vi "ROSSubscriber.vi"(2 "Response":T2, 3 "ROS":T3={"topic port"=1236, "Node"="/labview", "topic"="/robot/head/command_head_nod", "type"="std_msgs/Bool", "node port"=7000, "error "={"status"=FALSE, "code"=0, "source"=""}, "Direction"=enum."Publisher", "Update (ms)"=1, "FIFO size"=1}) -> ()   [LabVIEW 2015]
uses:
  SubVIs/_ROSControl.ctl
  SubVIs/_ROSDirection.ctl
  Console/Servers/ServerSubs/ROSLog.ctl
  _ROSDefinition.vi
panel:
  out "publishers":T1(array[cluster])
  out "Queue log":string
  out "read":string
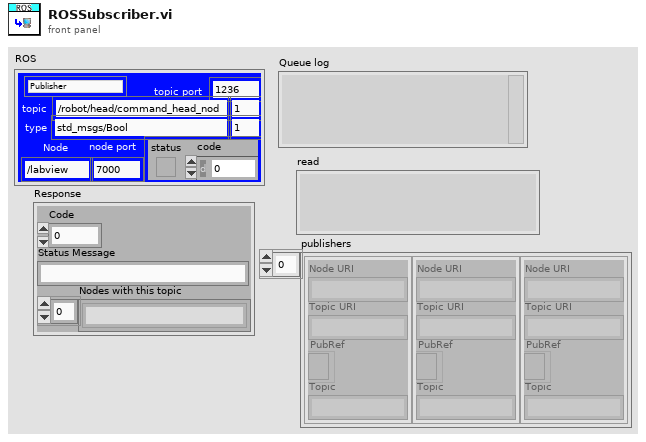
[diagram p1: front panel]
types:
  T1 = cluster{"Node URI":string, "Topic URI":string, "PubRef":refnum<k5>, "Topic":string}[]
  T2 = cluster{"Code":i32, "Status Message":string, "Nodes with this topic":string[]}
  T3 = typedef "_ROSControl.ctl" = cluster{"topic port":u16, "Node":string, "topic":string, "type":string, "node port":u16, "error ":errorcluster, "Direction":T4, "Update (ms)":u16, "FIFO size":u16}
  T4 = typedef "_ROSDirection.ctl" = enum16{"Node", "Publisher", "Subscriber", "ServiceClient", "ServiceProvider"}
  T5 = enum16{"Reset Log", "Add Client", "Remove Client", "Add Task"}
  T6 = cluster{"Node URI":string, "Topic URI":string, "PubRef":refnum<k5>, "Topic":string}
  T7 = typedef "ROSLog.ctl" = cluster{"Sent":string, "Reply":string, "MethodName":string, "success":bool, "Dir1":string, "Dir2":string, "Time Stamp":string, "error":errorcluster, "Preamble":string, "Midamble":string, "Postamble":string}
  T8 = cluster{"Caller ID":string, "Topic Name":string, "Node URIs":string[]}
  T9 = cluster{"Protocol":string, "Code":i32, "IP":string, "Port":i32}
  T10 = cluster{"Protocol":string, "Topic URI":string, "PubRef":refnum<k5>, "topic":string}
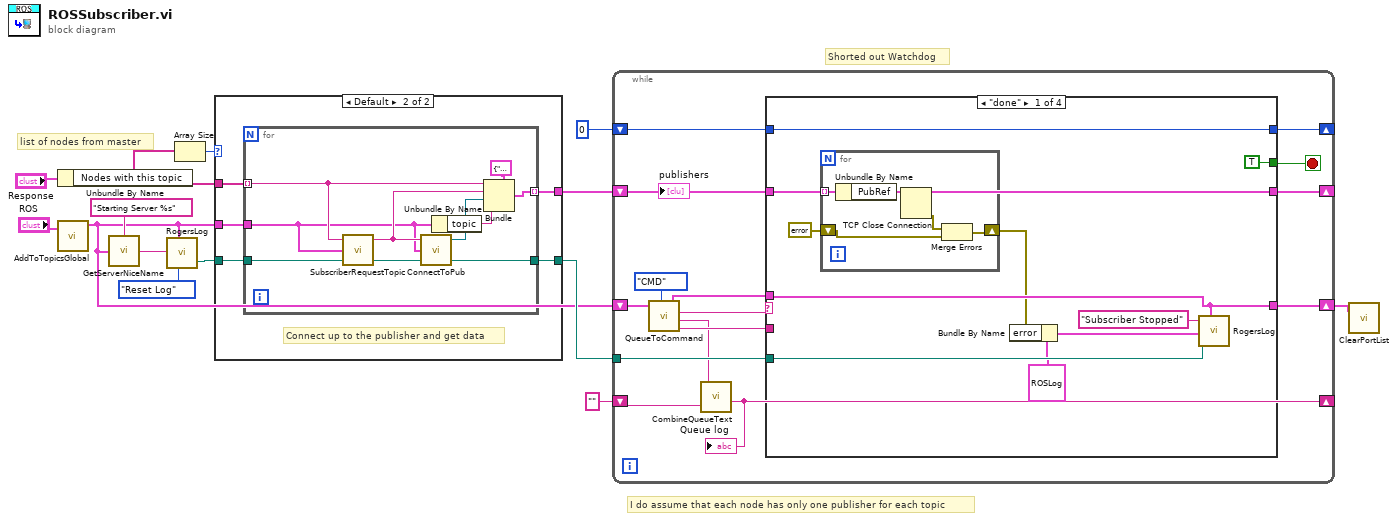
[diagram p0: block diagram]
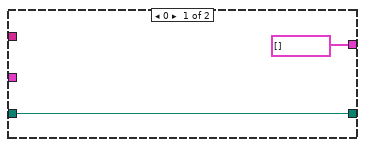
[diagram p2: hidden frame]
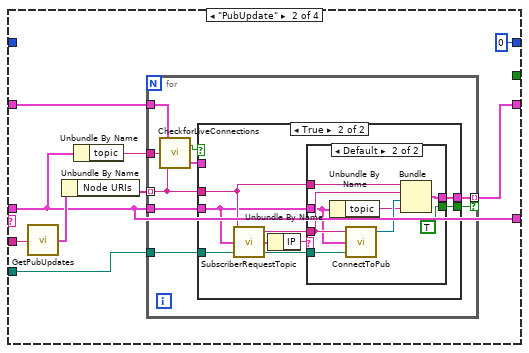
[diagram p3: hidden frame]
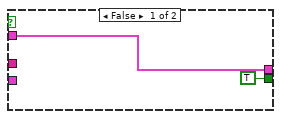
[diagram p4: hidden frame]
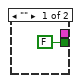
[diagram p5: hidden frame]
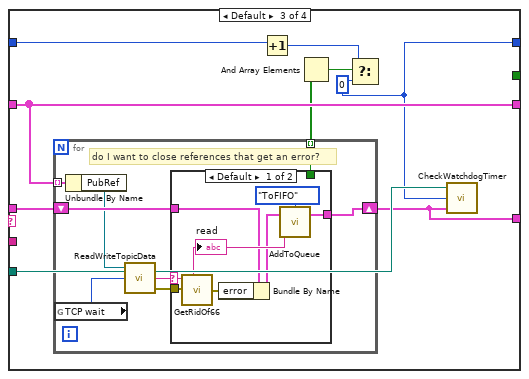
[diagram p6: hidden frame]
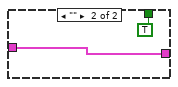
[diagram p7: hidden frame]
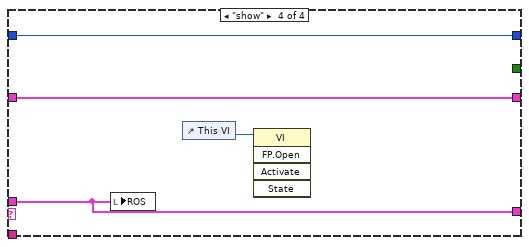
[diagram p8: hidden frame]
diagram:
  # "Shorted out Watchdog"
  # "I do assume that each node has only one publisher for each topic"
  # "list of nodes from master"
  n1 = Unbundle By Name("Response") -> ("Nodes with this topic"=w6:string[])
  n2 = call "AddToTopicsGlobal.vi"("ROS in"="ROS") -> ("ROS out"=w1:T3)  [unwired: 2 in]
  n3 = call "GetServerNiceName.vi"("ROS"=w1, "Text to add"="Starting Server %s") -> ("String"=w11:string)
  n4 = call "RogersLog.vi"("Text to add"=w11, "ROS"=w1, "Task"=T5."Reset Log") -> ("LogPath out"=w9:path)  [unwired: 2 in, 1 out]
  n5 = Array Size(array=w6) -> (size(s)=w5:i32)
  n6 = case shown="Default" w5 {
    tunnel: w6 -> [_ w21]
    tunnel: [T1 [] w20] -> w13
    tunnel: w9 -> [w15 w19]
    tunnel: w1 -> [_ w18]
    tunnel: [w15 w17] -> w8
    frame 0 {
    }
    frame Default {
      # "Connect up to the publisher and get data"
      n7 = for {
        tunnel: w21 -> [w28] mode=indexing
        tunnel: [w25] -> w20 mode=indexing
        tunnel: w19 -> [w31]
        tunnel: w18 -> [w23]
        tunnel: [w29] -> w17
        n8 = call "SubscriberRequestTopic.vi"("LogPath in"=w31, "ROS"=w23, "Node URI"=w28) -> ("LogPath out"=w30:path, "Topic URI"=w27:string)  [unwired: 1 out]
        n9 = call "ConnectToPub.vi"("LogPath in"=w30, "ROS"=w23, "IP"=w27) -> ("LogPath out"=w29:path, "PubRef"=w26:refnum<k5>)  [unwired: 1 out]
        n10 = Unbundle By Name(w23) -> ("topic"=w22:string)
        n11 = Bundle(cluster=T6 {"Node URI"="", "Topic URI"="", "PubRef"=refnum, "Topic"=""} ("output cluster"), "Node URI"=w28, "Topic URI"=w27, "PubRef"=w26, "Topic"=w22) -> (w25:T6)
      }
    }
  }
  n12 = while {
    shift-right: [w42] -> _
    shift-left: w13 -> [w46]
    tunnel: w8 -> [w41]
    shift-right: [w39] -> _
    shift-left: 0 -> [w40]
    shift-right: [w36] -> _
    shift-left: "" ("New List") -> [w38]
    shift-right: [w33] -> w3
    shift-left: w1 -> [w35]
    stop <- w44 stop-if-true
    n13 = call "QueueToCommand.vi"("ROS"=w35, "Check"=enum16{"Cmd+Write", "FIFO", "CMD", "CMD /wait"}."CMD") -> ("ROS out"=w34:T3, "Command"=w45:string, "Queue log"=w37:string, "data"=w43:string)  [unwired: 1 in]
    n14 = call "CombineQueueText.vi"("Old List"=w38, "Queue In"=w37) -> ("New List"=w36:string)  [unwired: 1 in]
    "Queue log" <- w36
    n15 = case shown="\"done\"" w45 {
      tunnel: w46 -> [w55 w64 w108 w129]
      tunnel: [TRUE _ _ _] -> w44
      tunnel: w43 -> [_ w68 _ _]
      tunnel: [w55 w65 w108 w129] -> w42
      tunnel: w34 -> [w51 w62 w101 w126]
      tunnel: w41 -> [w53 w66 w103 _]
      tunnel: w40 -> [w52 _ w104 w127]
      tunnel: [w52 0 w102 w127] -> w39
      tunnel: [w51 w62 w100 w126] -> w33
      frame "done" {
        n16 = for {
          tunnel: w55 -> [w61] mode=indexing
          shift-right: [w57] -> w48
          shift-left: errorcluster {"status"=FALSE, "code"=0, "source"=""} ("error IO") -> [w58]
          n17 = Unbundle By Name(w61) -> ("PubRef"=w60:refnum<k5>)
          n18 = TCP Close Connection(connection ID=w60) -> (error out=w59:errorcluster)  [unwired: 2 in, 1 out]
          n19 = Merge Errors(w59, w58) -> (w57:errorcluster)
        }
        n20 = Bundle By Name(cluster=T7 {"Sent"="", "Reply"="", "MethodName"="", "success"=TRUE, "Dir1"="", "Dir2"="", "Time Stamp"="", "error"={"status"=FALSE, "code"=0, "source"=""}, "Preamble"="", "Midamble"="", "Postamble"=""} ("Log"), "error"=w48) -> (w47:T7)
        n21 = call "RogersLog.vi"("Text to add"="Subscriber Stopped", "ROS"=w51, "Log"=w47, "LogPath in"=w53) -> ()  [unwired: 1 in, 2 out]
      }
      frame "PubUpdate" {
        n22 = call "GetPubUpdates.vi"("XML"=w68) -> ("PubUpdate"=w69:T8)
        n23 = Unbundle By Name(w69) -> ("Node URIs"=w67:string[])
        n24 = Unbundle By Name(w62) -> ("topic"=w63:string)
        n25 = for {
          tunnel: w67 -> [w75] mode=indexing
          tunnel: w66 -> [w79]
          tunnel: w62 -> [w78]
          tunnel: [w77] -> w65 mode=indexing if=w71
          tunnel: w64 -> [w76]
          tunnel: w63 -> [w72]
          n26 = call "CheckforLiveConnections.vi"("Node URI"=w75, "topic"=w72, "Connections"=w76) -> ("Connection"=w73:T6, "new?"=w74:bool)
          n27 = case shown="True" w74 {
            tunnel: w79 -> [_ w90]
            tunnel: w78 -> [_ w85]
            tunnel: w75 -> [_ w88]
            tunnel: [w81 w86] -> w77
            tunnel: w73 -> [w81 _]
            tunnel: [TRUE w82] -> w71
            frame False {
            }
            frame True {
              n28 = call "SubscriberRequestTopic.vi"("LogPath in"=w90, "ROS"=w85, "Node URI"=w88) -> ("LogPath out"=w89:path, "Topic Request Reply"=w84:T9, "Topic URI"=w87:string)
              n29 = Unbundle By Name(w84) -> ("IP"=w83:string)
              n30 = case shown="Default" w83 {
                tunnel: w89 -> [_ w99]
                tunnel: w88 -> [_ w98]
                tunnel: w87 -> [_ w97]
                tunnel: [_ w95] -> w86
                tunnel: w85 -> [_ w93]
                tunnel: [FALSE TRUE] -> w82
                frame "" {
                }
                frame Default {
                  n31 = Unbundle By Name(w93) -> ("topic"=w94:string)
                  n32 = call "ConnectToPub.vi"("LogPath in"=w99, "ROS"=w93, "IP"=w97) -> ("PubRef"=w96:refnum<k5>)  [unwired: 2 out]
                  n33 = Bundle("Protocol"=w98, "Topic URI"=w97, "PubRef"=w96, "topic"=w94) -> (w95:T10)  [unwired: 1 in]
                }
              }
            }
          }
        }
      }
      frame Default {
        w102 = 0
        n34 = for {
          tunnel: w108 -> [w112] mode=indexing
          tunnel: [w113] -> w107 mode=indexing
          shift-right: [w110] -> w100
          shift-left: w101 -> [w114]
          # "do I want to close references that get an error?"
          n35 = global read "_ROSDefinition.vi" "TCP wait"() -> (w109:i32)
          n36 = Unbundle By Name(w112) -> ("PubRef"=w111:refnum<k5>)
          n37 = call "ReadWriteTopicData.vi"("timeout ms (1000)"=w109, "connection ID in"=w111) -> ("error out"=w115:errorcluster, "data out"=w116:string)  [unwired: 1 in, 1 out]
          n38 = case shown="Default" w116 {
            selector: w116 -> [w123 _]
            tunnel: w114 -> [w121 w124]
            tunnel: w115 -> [w118 _]
            tunnel: [_ TRUE] -> w113
            tunnel: [w119 w124] -> w110
            frame Default {
              n39 = call "GetRidOf66.vi"("error in (no error)"=w118) -> ("error out"=w117:errorcluster)
              n40 = Bundle By Name(cluster=w121, "error"=w117) -> (w120:T3)
              n41 = call "AddToQueue.vi"("Cmd"=w123, "ROS"=w120, "Type"=enum16{"topic", "node", "ToFIFO"}."ToFIFO") -> ("ROS out"=w119:T3)  [unwired: 2 in]
              "read" <- w123
            }
            frame "" {
            }
          }
        }
        n42 = Increment(x=w104) -> (x+1=w105:i32)
        n43 = And Array Elements(Boolean array=w107) -> (logical AND=w106:bool)
        n44 = Select(t=w105, s=w106, f=w102) -> ()  [unwired: 1 out]
        n45 = call "CheckWatchdogTimer.vi"("ROS"=w100, "itteration"=w102, "LogPath in"=w103) -> ()  [unwired: 3 in]
      }
      frame "show" {
        n46 = local write "ROS"(w126) -> ()
        n47 = control-ref of="This VI"() -> (w128:refnum<vi>)
        n48 = invoke class="VI" method="FP.Open"(reference=w128) -> ()  [unwired: 4 in, 5 out]
      }
    }
    "publishers" <- w46
  }
  n49 = call "ClearPortList.vi"("ROS"=w3) -> ()  [unwired: 2 in]
